vi "Online Noise Reduction.vi"() -> ()   [LabVIEW 2023]
doc: "This example shows the application of linear Time Frequency Analysis VIs in online noise reduction. \n\nFor nonstationary signals whose spectral contents evolve over time, you usually use time-varying filters to reduce noise in the signals. The specification of a time-varying filter changes over time and is adaptable to signals. One typical implementation of the time-varying filter consists of the following three steps: converting a signal into the time-frequency representation using the Gabor transform, removing noise in the time-frequency domain, and reconstructing the signal with noise reduced using the Gabor expansion. \n\nThis example uses the TFA Online Gabor Transform VI to convert a time-domain signal into the time-frequency representation, sets the Gabor coefficients whose magnitude is smaller than a threshold to zero, and uses the TFA Online Gabor Expansion VI to reconstruct the time-domain signal with noise reduced. \n\n<b>Instructions:</b>\n1) Run this VI.\n2) Compare the <b>Noisy Signal</b> and <b>Denoised signal</b>.\n3) Browse the Block Diagram to learn how to implement online noise reduction application with the TFA Online Gabor Transform VI and the TFA Online Gabor Expansion VI."
uses:
  Instance           8 30Saved   Online Noise Reduction .vi
  <vilib>/addons/Time Frequency Analysis/Transform.llb/TFA Online Gabor Transform (Real).vi
  <vilib>/addons/Time Frequency Analysis/Transform.llb/TFA Online Gabor Expansion (Real).vi
  <vilib>/addons/_Advanced Signal Processing/NI_AdvSigProcTFA.lvlib
  <vilib>/Analysis/NI_AALBase.lvlib
panel:
  out "aspt-left-top":bool
  out "Denoised Signal":dbl[](graph)
  out "Gabor Coefficients after Thresholding":dbl[][](graph)
  out "Magnitude of Gabor Coefficients":dbl[][](graph)
  out "Noisy Signal":dbl[](graph)
  in  "Threshold":dbl=6.0 step=0.1 format="%.1f"
  in  "Stop":bool
  # "Overview: Shows the application of linear Time Frequency Analysis VIs in online noise reduction.\nRequirements: LabVIEW Full Development System, Advanced Signal Processing Toolkit\nInstructions: \n1. Run this VI.\n2. Compare the Noisy Signal and Denoised signal.\n3. Browse the block diagram to learn how to implement online noise reduction application with the TFA Online Gabor Transform VI and the TFA Online Gabor Expansion VI.\n4. Click Stop to stop the VI."
  # "Processing in Time-Frequency Domain"
  # "Time Domain"
  # "Time Domain"
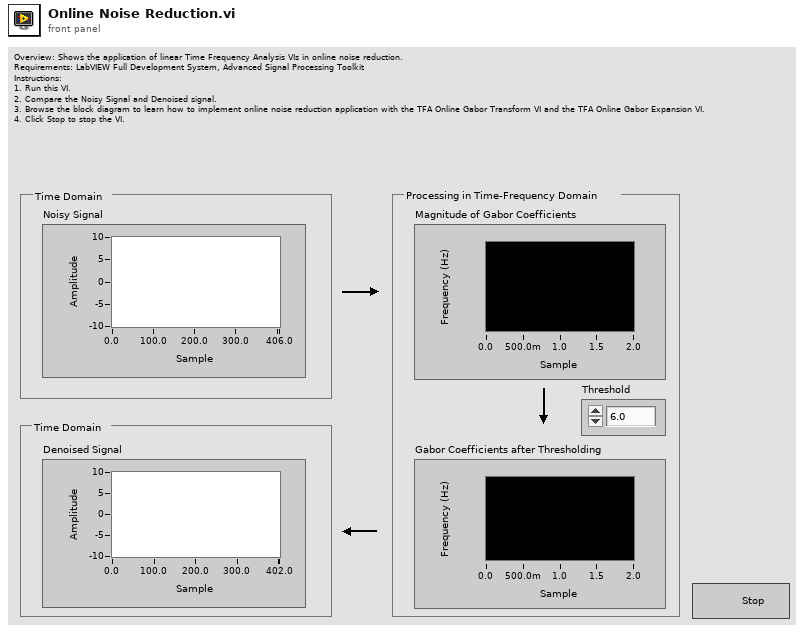
[diagram p1: front panel]
types:
  T1 = cluster{"synthesis window":dbl[], "dM (time steps)":i32, "N (frequency bins)":i32}
  T2 = cluster{"analysis window":dbl[], "dM (time steps)":i32, "N (frequency bins)":i32}
  T3 = cluster{"frequency offset":dbl, "frequency multiplier":dbl}
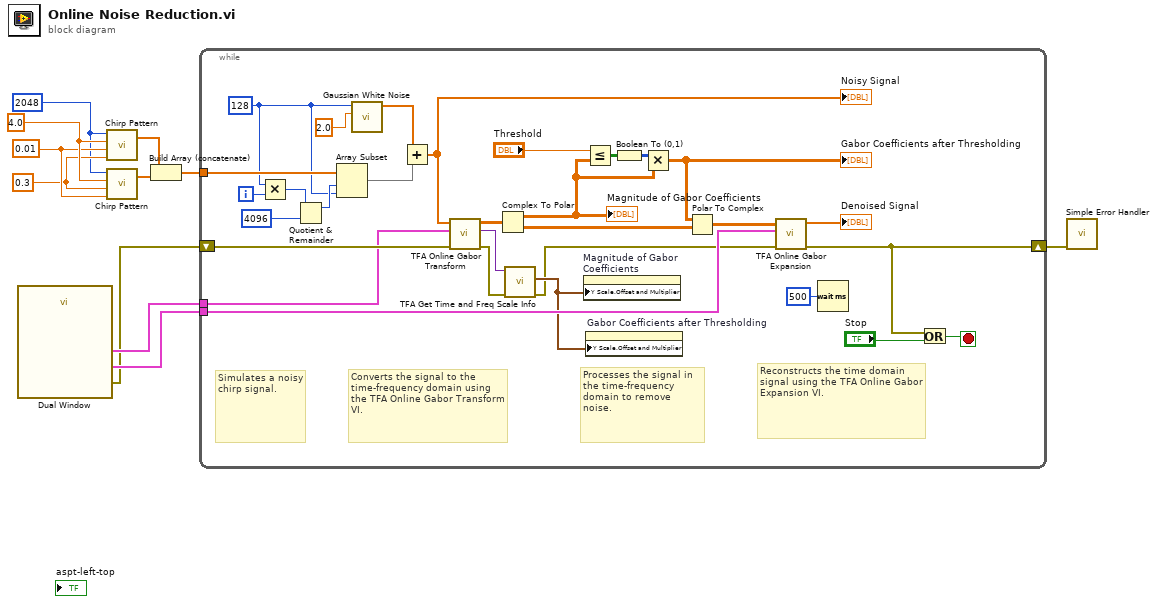
[diagram p0: block diagram]
diagram:
  w6 = 2048 ("samples")
  w11 = 4.0 ("amplitude")
  w9 = 0.3 ("f2")
  w10 = 0.01 ("f1")
  n1 = call "Dual Window"() -> ("error out"=w2:errorcluster, "expansion info"=w3:T1, "transform info"=w4:T2)  [unwired: 1 in, 8 out]
  n2 = call <vilib>:"Chirp Pattern.vi"("f2"=w9, "f1"=w10, "amplitude"=w11, "samples"=w6) -> ("Chirp Pattern"=w8:dbl[])  [unwired: 1 out]
  n3 = call <vilib>:"Chirp Pattern.vi"("f2"=w10, "f1"=w9, "amplitude"=w11, "samples"=w6) -> ("Chirp Pattern"=w7:dbl[])  [unwired: 1 out]
  n4 = Build Array (concatenate)(w8, w7) -> (w5:dbl[])
  n5 = while {
    tunnel: w4 -> [w32]
    tunnel: w3 -> [w31]
    shift-right: [w12] -> w1
    shift-left: w2 -> [w41]
    tunnel: w5 -> [w28]
    i -> [w27]
    stop <- w29 stop-if-true
    w21 = 128 ("samples")
    # "Reconstructs the time domain signal using the TFA Online Gabor Expansion VI."
    # "Converts the signal to the\ntime-frequency domain using the TFA Online Gabor Transform VI."
    # "Processes the signal in the time-frequency \ndomain to remove noise."
    # "Simulates a noisy chirp signal."
    n6 = Multiply(x=w21, y=w27) -> (x*y=w25:i32)
    n7 = Quotient & Remainder(x=w25, y=4096) -> (x-y*floor(x/y)=w24:i32)  [unwired: 1 out]
    n8 = Array Subset(array=w28, index=w24, length=w21) -> (w22:dbl[])
    n9 = call <vilib>:"Gaussian White Noise.vi"("standard deviation"=2.0, "samples"=w21) -> ("Gaussian noise pattern"=w23:dbl[])  [unwired: 8 in, 1 out]
    n10 = Add(x=w23, y=w22) -> (x+y=w34:dbl[])
    "Noisy Signal" <- w34
    n11 = call-poly <vilib>:"TFA Online Gabor Transform.vi"("error in (no error)"=w41, "transform info"=w32, "signal"=w34) -> ("error out"=w14:errorcluster, "scale info"=w17:variant, "Gabor coef"=w19:cdb[][])  [unwired: 6 out]
    n12 = Complex To Polar(r * e^(i*theta)=w19) -> (r=w18:dbl[][], theta=w37:dbl[][])
    "Magnitude of Gabor Coefficients" <- w18
    n13 = call <vilib>:"TFA Get Time and Freq Scale Info.vi"("error in (no error)"=w14, "scale info"=w17) -> ("error out"=w13:errorcluster, "frequency info"=w16:T3)  [unwired: 8 out]
    n14 = property on="Magnitude of Gabor Coefficients" class="IntChart (strict)"("Y Scale.Offset and Multiplier"=w16) -> ()  [unwired: 2 in, 2 out]
    n15 = Less Or Equal?(x="Threshold", y=w18) -> (x <= y?=w39:bool[][])
    n16 = property on="Gabor Coefficients after Thresholding" class="IntChart (strict)"("Y Scale.Offset and Multiplier"=w16) -> ()  [unwired: 2 in, 2 out]
    n17 = Boolean To (0,1)(Boolean=w39) -> (0, 1=w38:i16[][])
    n18 = Multiply(x=w38, y=w18) -> (x*y=w20:dbl[][])
    "Gabor Coefficients after Thresholding" <- w20
    n19 = Polar To Complex(1:w37, 2:w20) -> (0:w36:cdb[][])
    n20 = call-poly <vilib>:"TFA Online Gabor Expansion.vi"("error in (no error)"=w13, "expansion info"=w31, "Gabor coef"=w36) -> ("error out"=w12:errorcluster, "signal"=→"Denoised Signal":dbl[])  [unwired: 7 out]
    n21 = Wait (ms)(milliseconds to wait=u32 500 ("millisecond multiple")) -> ()  [unwired: 1 out]
    n22 = Or(x=w12, y="Stop") -> (x .or. y?=w29:bool)
  }
  n23 = call <vilib>:"Simple Error Handler.vi"("error in (no error)"=w1) -> ()  [unwired: 1 in, 8 out]
